vi "Test Temperature.vi"(8 "error in (no error)":errorcluster, 11 "Instrument.Cryostat in":refnum<class "Instrument.Cryostat.lvclass">) -> (0 "error out":errorcluster, 3 "Instrument.Cryostat out":refnum<class "Instrument.Cryostat.lvclass">)   [LabVIEW 2016, in "Instrument.Cryostat.lvclass"]
uses:
  Instrument.Cryostat.lvclass
  <vilib>/addons/_JKI Toolkits/Caraya/classes/Assert/Assert.lvclass
  <vilib>/addons/_JKI Toolkits/Caraya/classes/Test/Test.lvclass
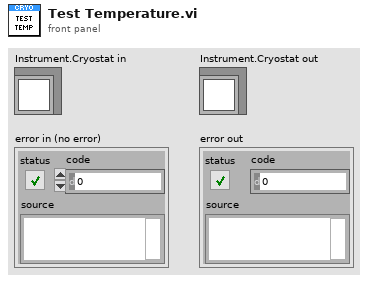
[diagram p1: front panel]
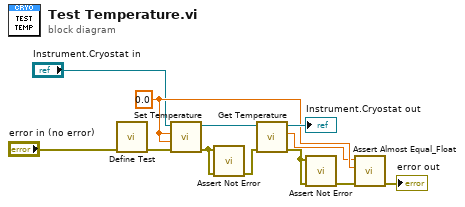
[diagram p0: block diagram]
diagram:
  w5 = 0.0 ("Angle (°)")
  n1 = call <vilib>:"Define Test.vi"("error in (no error)"="error in (no error)") -> ("error out"=w1:errorcluster)  [unwired: 10 in]
  n2 = call-dynamic "Set Temperature.vi"("error in (no error)"=w1, "Rate (K/min)"=w5, "Temperature (K)"=w5, "Instrument.Cryostat in"="Instrument.Cryostat in") -> ("error out"=w8:errorcluster, "Instrument.Cryostat out"=w6:refnum<class "Instrument.Cryostat.lvclass">)  [unwired: 6 in]
  n3 = call <vilib>:"Assert Not Error.vi"("error in (no error)"=w8, "Not Error?"=w8) -> ("error out"=w9:errorcluster)  [unwired: 9 in]
  n4 = call-dynamic "Get Temperature.vi"("error in (no error)"=w9, "Instrument.Cryostat in"=w6) -> ("error out"=w10:errorcluster, "Temperature (K)"=w4:dbl, "Instrument.Cryostat out"=→"Instrument.Cryostat out":refnum<class "Instrument.Cryostat.lvclass">)  [unwired: 6 in, 1 out]
  n5 = call <vilib>:"Assert Not Error.vi"("error in (no error)"=w10, "Not Error?"=w10) -> ("error out"=w11:errorcluster)  [unwired: 9 in]
  n6 = call <vilib>:"Assert Almost Equal_Float.vi"("error in (no error)"=w11, "Y"=w5, "X"=w4) -> ("error out"=→"error out":errorcluster)  [unwired: 8 in]
